vi "1_maximum_acceleration_main.vi"() -> ()   [LabVIEW 2019]
uses:
  Shared VIs/TypeDef_TDMS_States.ctl
  <vilib>/myRIO/Common/Instrument Driver Framework/myRIO v1.0/Encoder/typedefs/Encoder Signal Mode.ctl
  <vilib>/myRIO/Instrument Drivers/Onboard IO/AI/typedefs/AI Reference.ctl
  <vilib>/myRIO/Common/Instrument Driver Framework/Utilities/typedefs/myRIO Generic Hardware Reference.ctl
  <vilib>/myRIO/Common/Instrument Driver Framework/Utilities/typedefs/Hardware Version Enum.ctl
  <vilib>/myRIO/Common/Instrument Driver Framework/Utilities/typedefs/myRIO v1.0 Reference.ctl
  <vilib>/myRIO/Common/Instrument Driver Framework/Utilities/typedefs/Generic FPGA Reference.ctl
  <vilib>/myRIO/Common/Instrument Driver Framework/myRIO v1.0/AI/typedefs/AI Channels List.ctl
  <vilib>/myRIO/Common/Instrument Driver Framework/myRIO v1.0/AI/typedefs/AI Channels Enum.ctl
  <vilib>/myRIO/Common/Instrument Driver Framework/Utilities/typedefs/Analog Scaling Constants List.ctl
  <vilib>/myRIO/Common/Instrument Driver Framework/Utilities/typedefs/Analog Scaling Constants.ctl
  <vilib>/userDefined/High Color/nirio_resource_hc.ctl
  <vilib>/myRIO/Instrument Drivers/Onboard IO/AO/typedefs/AO Reference.ctl
  <vilib>/myRIO/Common/Instrument Driver Framework/myRIO v1.0/AO/typedefs/AO Channels List.ctl
  <vilib>/myRIO/Common/Instrument Driver Framework/myRIO v1.0/AO/typedefs/AO Channels Enum.ctl
  <vilib>/Platform/TimedLoop/XDataNode/timing_clust.ctl
  <vilib>/Platform/TimedLoop/XDataNode/nitl_modes.ctl
  <vilib>/Platform/TimedLoop/XDataNode/wakeup.ctl
  <vilib>/myRIO/Common/Instrument Driver Framework/myRIO v1.0/AI/vis/myRIO v1.1 Open AI.vi
  <vilib>/myRIO/Common/Instrument Driver Framework/myRIO v1.0/AO/vis/myRIO v1.1 Open AO.vi
  <vilib>/myRIO/Common/Instrument Driver Framework/Utilities/vis/Validate Channels.vi
  <vilib>/myRIO/Common/Instrument Driver Framework/myRIO v1.0/AI/vis/myRIO v1.0 Reserve AI.vi
  <vilib>/myRIO/Common/Instrument Driver Framework/myRIO v1.0/AO/vis/myRIO v1.0 Reserve AO.vi
  <vilib>/myRIO/Common/Instrument Driver Framework/myRIO v1.0/AI/vis/myRIO v1.0 Close AI.vi
  <vilib>/myRIO/Common/Instrument Driver Framework/myRIO v1.0/Encoder/vis/myRIO v1.0 Close Encoder.vi
  <vilib>/myRIO/Common/Instrument Driver Framework/myRIO v1.0/AO/vis/myRIO v1.0 Close AO.vi
  <vilib>/myRIO/Common/Instrument Driver Framework/myRIO v1.0/AI/vis/myRIO v1.0 Build MUX Configuration AI.vi
  <vilib>/myRIO/Common/Instrument Driver Framework/myRIO v1.0/Resource Manager/vis/myRIO v1.0 Reserve Channel List.vi
  <vilib>/myRIO/Common/Instrument Driver Framework/myRIO v1.0/AO/vis/myRIO v1.0 Build MUX Configuration AO.vi
  <vilib>/myRIO/Common/Instrument Driver Framework/myRIO v1.0/AI/vis/myRIO v1.0 Unreserve AI.vi
  <vilib>/myRIO/Common/Instrument Driver Framework/myRIO v1.0/Encoder/vis/myRIO v1.0 Unreserve Encoder.vi
  <vilib>/myRIO/Common/Instrument Driver Framework/myRIO v1.0/AO/vis/myRIO v1.0 Unreserve AO.vi
  <vilib>/myRIO/Common/Instrument Driver Framework/myRIO v1.0/Resource Manager/vis/myRIO v1.0 Reserve Channel.vi
  <vilib>/myRIO/Common/Instrument Driver Framework/myRIO v1.0/Resource Manager/vis/myRIO v1.0 Unreserve Channel.vi
  <vilib>/myRIO/Common/Instrument Driver Framework/myRIO v1.0/Resource Manager/vis/myRIO v1.0 Unreserve Channel List.vi
  <vilib>/myRIO/Common/Instrument Driver Framework/myRIO v1.0/Encoder/vis/myRIO v1.0 Build MUX Configuration Encoder.vi
  <vilib>/myRIO/Common/Instrument Driver Framework/myRIO v1.0/Resource Manager/vis/myRIO v1.0 Build Mutex Name.vi
  <vilib>/myRIO/Common/Instrument Driver Framework/myRIO v1.0/Resource Manager/vis/myRIO v1.0 Create Configuration List.vi
  <vilib>/Utility/VariantDataType/GetNumericInfo.vi
  <vilib>/Utility/error.llb/Error Cluster From Error Code.vi
  <vilib>/myRIO/Common/Instrument Driver Framework/myRIO v1.0/myRIO v1.1 Open.vi
  <vilib>/myRIO/Common/Instrument Driver Framework/myRIO v1.0/AO/vis/myRIO v1.0 Get Scaling Constants AO.vi
  <vilib>/myRIO/Common/Instrument Driver Framework/Utilities/vis/IO Manager.vi
  <vilib>/myRIO/Common/Instrument Driver Framework/Utilities/vis/Configuration Manager.vi
  <vilib>/myRIO/Common/Instrument Driver Framework/myRIO v1.0/myRIO v1.0 Close.vi
  <vilib>/myRIO/Common/Instrument Driver Framework/myRIO v1.0/AO/vis/myRIO v1.0 Write AO.vi
  <vilib>/myRIO/Common/Instrument Driver Framework/myRIO v1.0/AI/vis/myRIO v1.0 Get Scaling Constants AI.vi
  <vilib>/myRIO/Common/Instrument Driver Framework/myRIO v1.0/AI/vis/myRIO v1.0 Read AI.vi
  <vilib>/myRIO/Common/Instrument Driver Framework/myRIO v1.0/Encoder/vis/myRIO v1.0 Read Encoder.vi
  <vilib>/myRIO/Common/Instrument Driver Framework/myRIO v1.0/Encoder/vis/myRIO v1.0 Enable Encoder.vi
  <vilib>/myRIO/Common/Instrument Driver Framework/myRIO v1.0/Encoder/vis/myRIO v1.0 Shutdown Encoder.vi
  <vilib>/myRIO/Common/Instrument Driver Framework/myRIO v1.0/Resource Manager/vis/myRIO v1.0 Configure IO.vi
  <vilib>/myRIO/Instrument Drivers/Onboard IO/AO/vis/myRIO AO Open.xnode
  <vilib>/myRIO/Instrument Drivers/Onboard IO/AI/vis/myRIO AI Open.xnode
  <vilib>/Platform/TimedLoop/XDataNode/XDataNode.xnode
  <vilib>/myRIO/Instrument Drivers/Onboard IO/Encoder/Encoder.lvlib
  <vilib>/myRIO/Instrument Drivers/Onboard IO/AO/AO.lvlib
  <vilib>/Platform/TimedLoop/XDataNode/XDNodeRunTimeDep.lvlib
  <vilib>/myRIO/Instrument Drivers/Onboard IO/AI/AI.lvlib
panel:
  in  "TDMS Storage File Input":string
  out "TDMS States":T1
  in  "Save data?":bool
  in  "START":bool
  in  "Motor Input Voltage [V]":dbl
  out "Current (A)":dbl
  out "Loop Number (dt = 1 ms)":dbl
  in  "STOP":bool
  out "Elapsed Time (ms)":dbl
  out "Initial Time (ms)":dbl
  out "Encoder Position (deg)":dbl
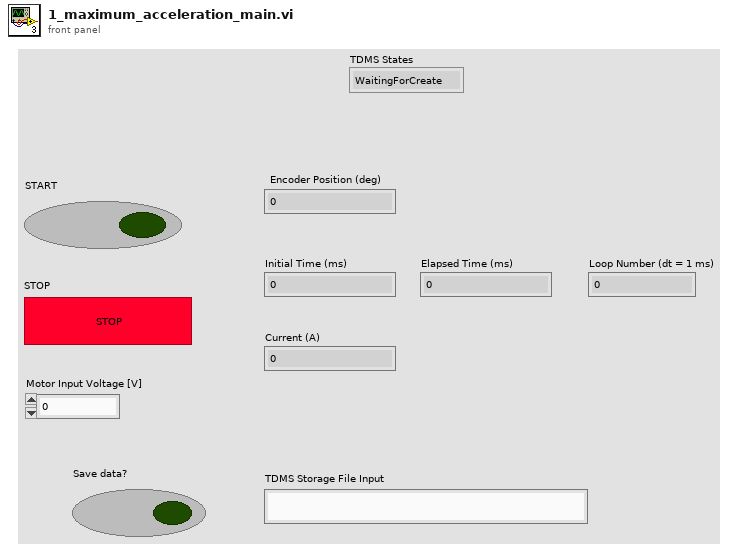
[diagram p1: front panel]
types:
  T1 = typedef "TypeDef_TDMS_States.ctl" = enum16{"WaitingForCreate", "Create", "Buffering", "Flushing", "Write", "Close"}
  T2 = typedef "nirio_resource_hc.ctl" = tag
  T3 = typedef "Hardware Version Enum.ctl" = enum16{"Unknown", "myRIO-1900", "myRIO-1950", "roboRIO", "NI ELVIS RIO CM", "ELVIS III"}
  T4 = enum16{"open", "open or create", "create or replace", "create", "open (read-only)"}
  T5 = typedef "XDNodeRunTimeDep.lvlib/timing_clust.ctl" = cluster{"Expected End [f-1]":u64, "Actual End [f-1]":u64, "Finished Late? [f-1]":bool, "Expected End [i-1]":u64, "Actual End [i-1]":u64, "Finished Late? [i-1]":bool, "Expected Start [i]":u64, "Actual Start [i]":u64, "Expected Start [f]":u64, "Actual Start [f]":u64, "Source Name":string, "Structure Name":string, "Period":i64, "Deadline":i64, "Offset":i64, "Start":i64, "Priority":i32, "Timeout":i32, "Mode":T6, "Wakeup Reason":T7, "Error":errorcluster, "Source Type":string, "Secondary Source Type":string, "Global End Time":u64, "Global Start Time":u64, "Frame Duration":u64, "Iteration Duration":u64, "Assigned CPU":i32, "I/O Scan Engine Mode":u32}
  T6 = typedef "XDNodeRunTimeDep.lvlib/nitl_modes.ctl" = enum32{"No Change", "Process missed periods, maintain original phase", "Discard missed periods, maintain original phase", "Process missed periods, ignore original phase", "Discard missed periods, ignore original phase"}
  T7 = typedef "XDNodeRunTimeDep.lvlib/wakeup.ctl" = enum32{"Normal", "Aborted", "Asynchronous wakeup", "Timing source error", "Timed loop error", "Timeout"}
  T8 = typedef "Encoder Signal Mode.ctl" = enum16{"Quadrature phase signal", "Step and direction signal"}
  T9 = typedef "AO.lvlib/AO Reference.ctl" = cluster{"myRIO Reference":T10, "AO Channel List":T13, "AO Scaling Constant List":T15}
  T10 = typedef "myRIO Generic Hardware Reference.ctl" = cluster{"myRIO Model":T3, "myRIO Hardware Reference":T11}
  T11 = typedef "myRIO v1.0 Reference.ctl" = cluster{"Generic FPGA Reference":T12, "Allow multiple opens":bool}
  T12 = typedef "Generic FPGA Reference.ctl" = refnum<k20>
  T13 = typedef "AO Channels List.ctl" = T14[]
  T14 = typedef "AO Channels Enum.ctl" = enum16{"Not Connected", "AudioOut/Left", "AudioOut/Right", "C/AO0", "C/AO1", "A/AO0", "A/AO1", "B/AO0", "B/AO1"}
  T15 = typedef "Analog Scaling Constants List.ctl" = T16[]
  T16 = typedef "Analog Scaling Constants.ctl" = cluster{"LSB Weight (Volts)":dbl, "Offset (Volts)":dbl, "Signed?":bool}
  T17 = typedef "AI.lvlib/AI Reference.ctl" = cluster{"myRIO Reference":T10, "AI Channels List":T18, "AI Scaling Constants List":T15}
  T18 = typedef "AI Channels List.ctl" = T19[]
  T19 = typedef "AI Channels Enum.ctl" = enum16{"Not Connected", "AudioIn/Left", "AudioIn/Right", "C/AI0", "C/AI1", "A/AI0", "A/AI1", "A/AI2", "A/AI3", "A/AI4", "A/AI5", "A/AI6", "A/AI7", "B/AI0", "B/AI1", "B/AI2", "B/AI3", "B/AI4", "B/AI5", "B/AI6", "B/AI7", "AI/AI0", "AI/AI1", "AI/AI2", "AI/AI3", "A/AI0 (DIFF)", "A/AI1 (DIFF)", "A/AI2 (DIFF)", "A/AI3 (DIFF)", "B/AI0 (DIFF)", "B/AI1 (DIFF)", "B/AI2 (DIFF)", "B/AI3 (DIFF)"}
  T20 = typedef "Encoder.lvlib/Encoder Reference.ctl" = cluster{"myRIO Reference":T10, "Encoder Channels Enum":T21}
  T21 = typedef "Encoder Channels Enum.ctl" = enum16{"Not Connected", "C/ENC0", "C/ENC1", "A/ENC", "A/ENC0", "A/ENC1", "A/ENC2", "A/ENC3", "A/ENC4", "A/ENC5", "A/ENC6", "A/ENC7", "A/ENC8", "A/ENC9", "B/ENC", "B/ENC0", "B/ENC1", "B/ENC2", "B/ENC3", "B/ENC4", "B/ENC5", "B/ENC6", "B/ENC7", "B/ENC8", "B/ENC9", "DIO/ENC0", "DIO/ENC1", "DIO/ENC2", "DIO/ENC3", "DIO/ENC4"}
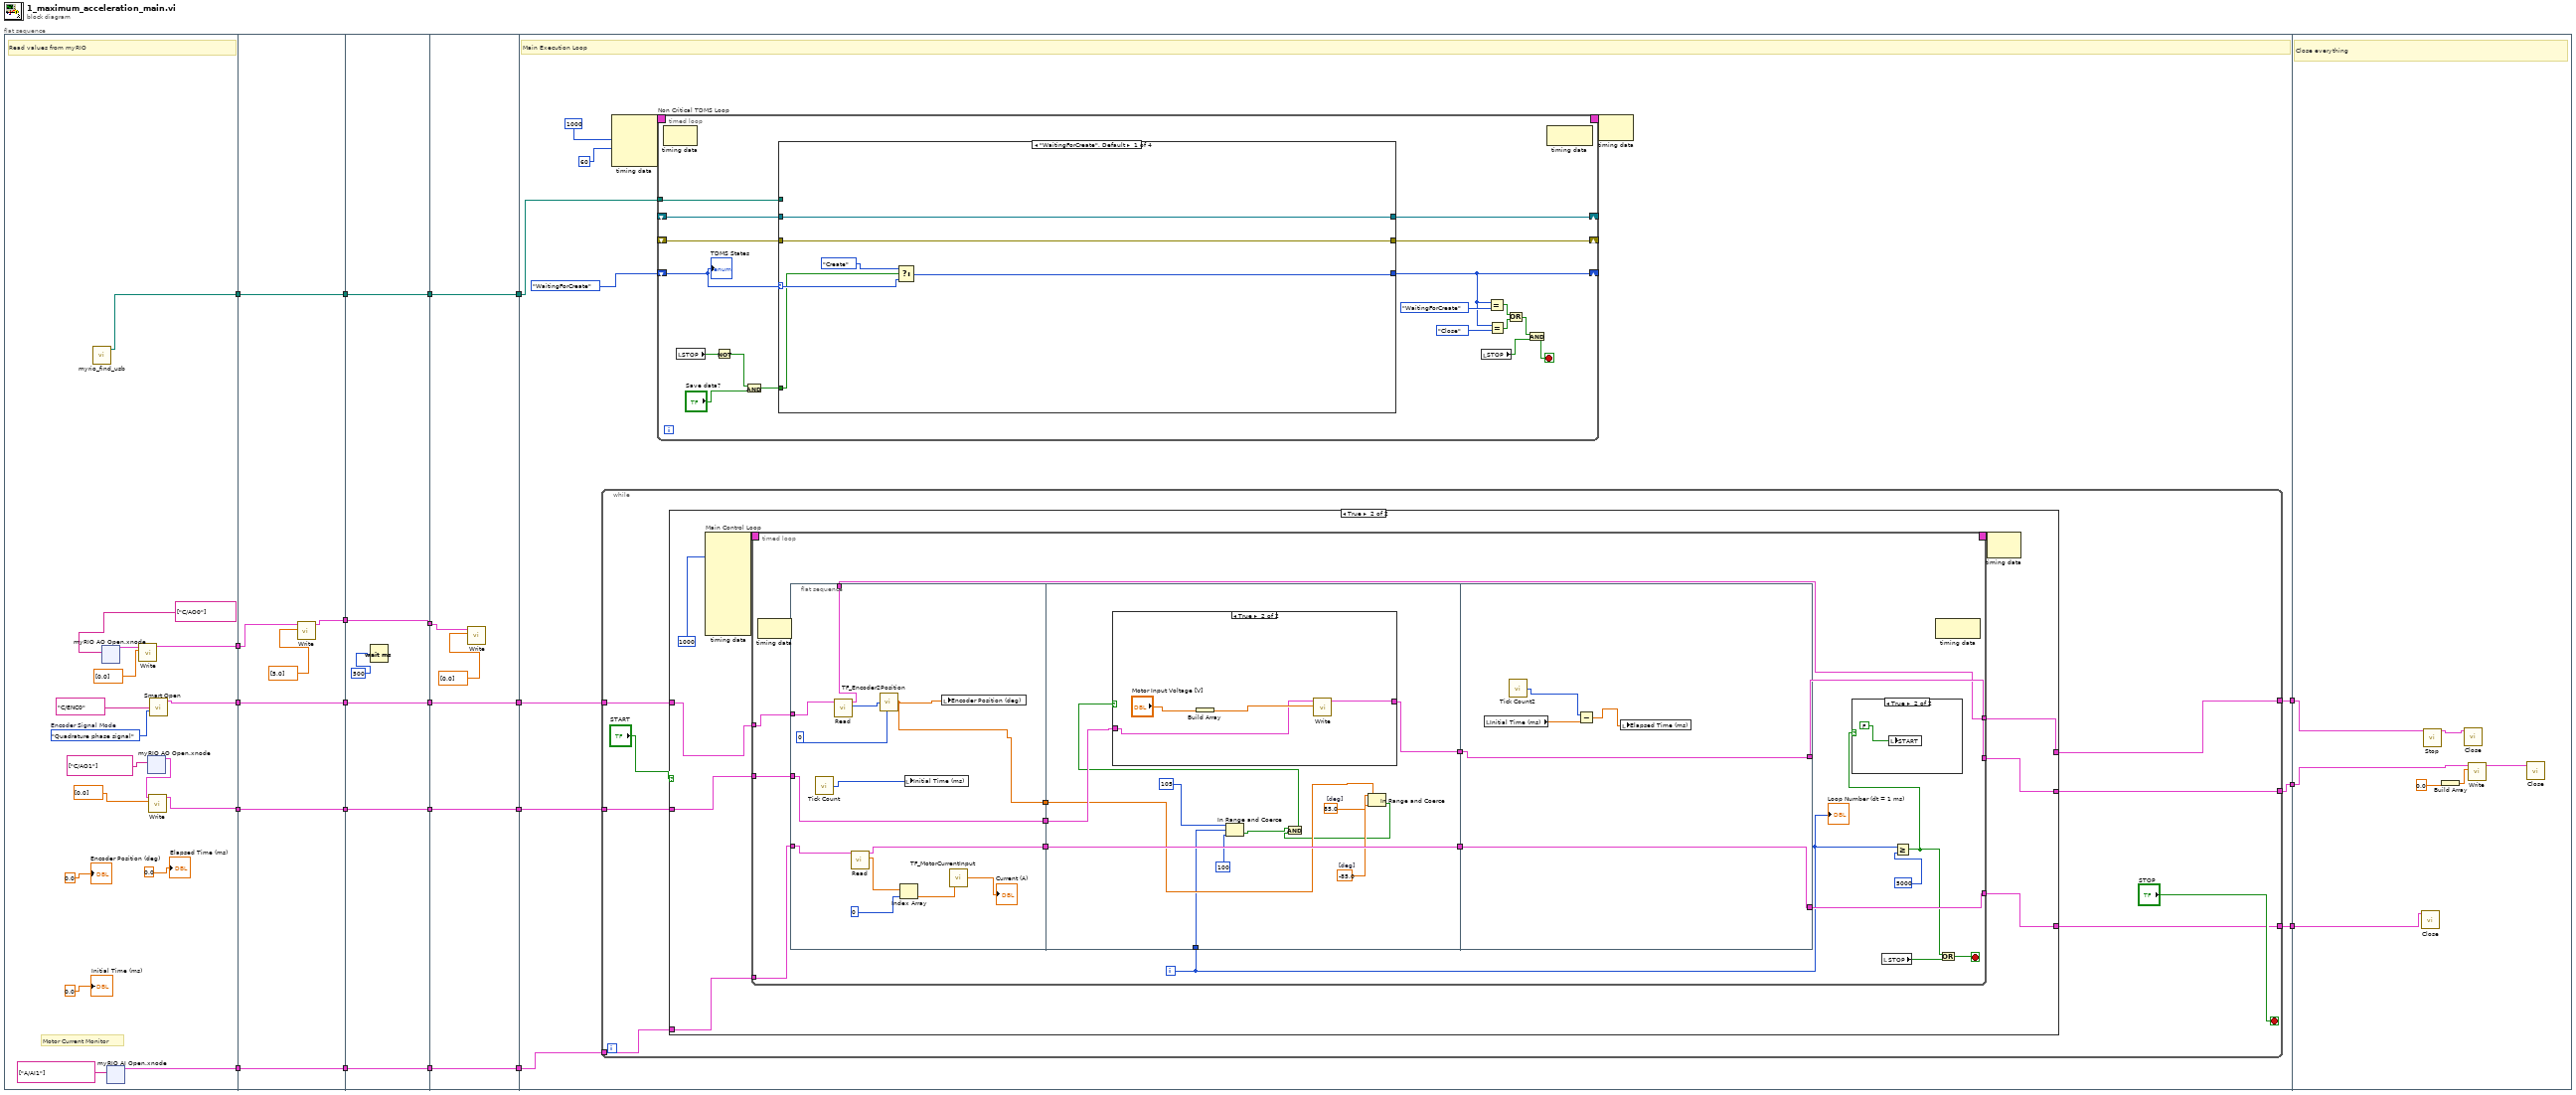
[diagram p0: block diagram]
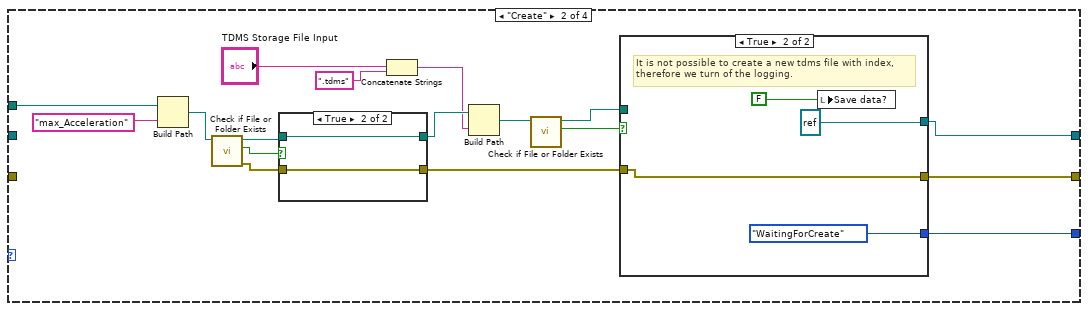
[diagram p2: hidden frame]
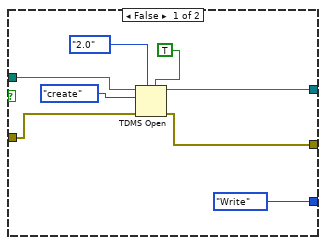
[diagram p3: hidden frame]
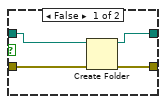
[diagram p4: hidden frame]
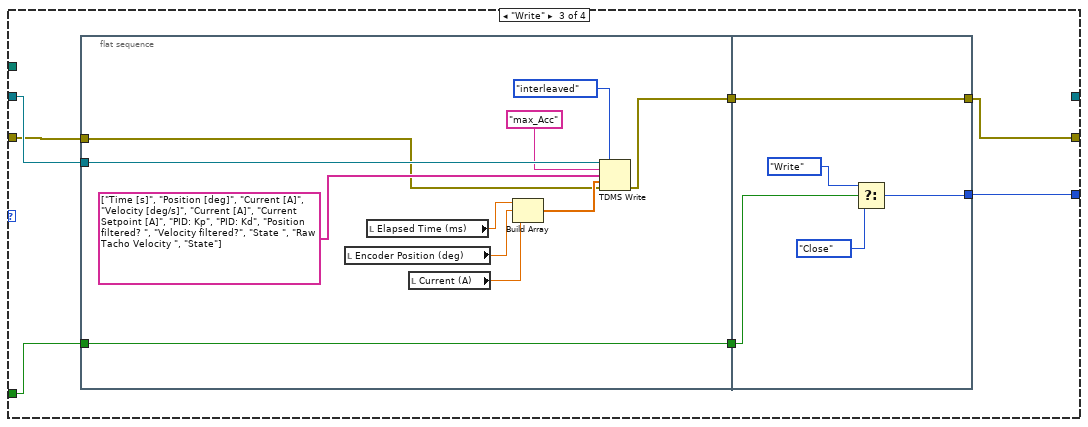
[diagram p5: hidden frame]
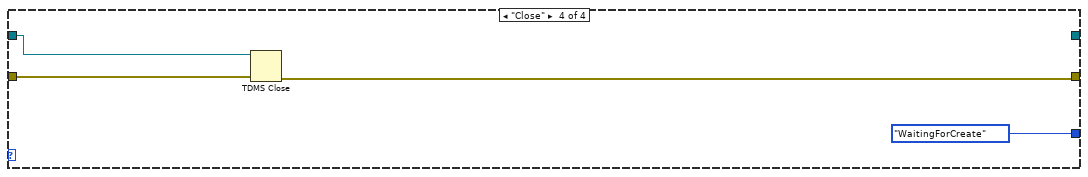
[diagram p6: hidden frame]
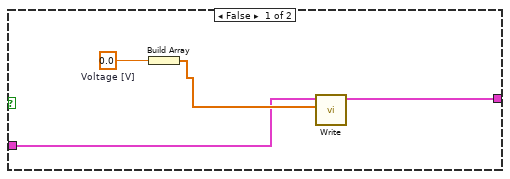
[diagram p9: hidden frame]
diagram:
  n1 = flat-sequence {
    tunnel: [w31] -> w15
    tunnel: [w30] -> w13
    tunnel: [w26] -> w11
    tunnel: [w24] -> w6
    tunnel: [w23] -> w1
    tunnel: w15 -> [w100]
    tunnel: [w100] -> w14
    tunnel: w13 -> [w99]
    tunnel: [w99] -> w12
    tunnel: w11 -> [w97]
    tunnel: [w96] -> w10
    tunnel: [w95] -> w7
    tunnel: w6 -> [w95]
    tunnel: [w94] -> w2
    tunnel: w1 -> [w94]
    tunnel: w14 -> [w106]
    tunnel: [w106] -> w20
    tunnel: w12 -> [w105]
    tunnel: [w105] -> w18
    tunnel: [w103] -> w16
    tunnel: w10 -> [w103]
    tunnel: [w102] -> w8
    tunnel: w7 -> [w102]
    tunnel: [w101] -> w3
    tunnel: w2 -> [w101]
    tunnel: w20 -> [w112]
    tunnel: [w112] -> w19
    tunnel: w18 -> [w111]
    tunnel: [w111] -> w17
    tunnel: w16 -> [w110]
    tunnel: [w108] -> w9
    tunnel: w8 -> [w108]
    tunnel: [w107] -> w4
    tunnel: w3 -> [w107]
    tunnel: w19 -> [w123]
    tunnel: w17 -> [w124]
    tunnel: [w121] -> w22
    tunnel: [w122] -> w21
    tunnel: w9 -> [w120]
    tunnel: [w119] -> w5
    tunnel: w4 -> [w113]
    tunnel: w22 -> [w301]
    tunnel: w21 -> [w300]
    tunnel: w5 -> [w299]
    frame #0 {
      w38 = Encoder_Signal_Mode."Quadrature phase signal"  # Encoder Signal Mode
      # "Motor Current Monitor"
      # "Read values from myRIO"
      n2 = call "myrio_find_usb.vi"() -> ("Largest USB Partition Path"=w23:path)  [unwired: 9 in, 2 out]
      n3 = xnode "myRIO AO Open.xnode"("Channel Names"=tag[] ["C/AO0"]) -> ("AO Ref Out"=w29:T9)  [unwired: 2 in, 1 out]
      n4 = xnode "myRIO AI Open.xnode"("Channel Names"=tag[] ["A/AI1"]) -> ("AI Ref Out"=w24:T17)  [unwired: 2 in, 1 out]
      n5 = call <vilib>:"Write.vi"("Values"=dbl[] [0.0], "AO Ref In"=w29) -> ("AO Ref Out"=w26:T9)  [unwired: 7 in, 1 out]
      n6 = xnode "myRIO AO Open.xnode"("Channel Names"=tag[] ["C/AO1"]) -> ("AO Ref Out"=w36:T9)  [unwired: 2 in, 1 out]
      n7 = call <vilib>:"Write.vi"("Values"=dbl[] [0.0], "AO Ref In"=w36) -> ("AO Ref Out"=w30:T9)  [unwired: 7 in, 1 out]
      n8 = call <vilib>:"Smart Open.vi"("Encoder Signal Mode"=w38, "Channel Name"=tag "C/ENC0") -> ("Encoder Ref Out"=w31:T20)  [unwired: 8 in, 1 out]
      "Encoder Position (deg)" <- 0.0
      "Initial Time (ms)" <- 0.0
      "Elapsed Time (ms)" <- 0.0
    }
    frame #1 {
      n9 = call <vilib>:"Write.vi"("Values"=dbl[] [5.0], "AO Ref In"=w97) -> ("AO Ref Out"=w96:T9)  [unwired: 7 in, 1 out]
    }
    frame #2 {
      n10 = Wait (ms)(milliseconds to wait=500) -> ()  [unwired: 1 out]
    }
    frame #3 {
      n11 = call <vilib>:"Write.vi"("Values"=dbl[] [0.0], "AO Ref In"=w110) -> ()  [unwired: 7 in, 2 out]
    }
    frame #4 {
      # "Main Execution Loop"
      n12 = while {
        tunnel: w124 -> [w225]
        tunnel: w123 -> [w224]
        tunnel: [w221] -> w122
        tunnel: [w222] -> w121
        tunnel: w120 -> [w220]
        tunnel: [w219] -> w119
        stop <- "STOP" stop-if-true
        n13 = case shown="True" "START" {
          tunnel: w225 -> [w227 w234]
          tunnel: w224 -> [w228 w233]
          tunnel: [w227 w232] -> w222
          tunnel: [w228 w231] -> w221
          tunnel: w220 -> [w226 w230]
          tunnel: [w226 w229] -> w219
          frame False {
          }
          frame True {
            n14 = node-c288(1000) -> (w237:T5)  [unwired: 9 in]
            n15 = timed-loop "Main Control Loop" {
              timing: w237 -> [_]
              timing-out: [_] -> w236
              tunnel: w233 -> [w253]
              tunnel: w234 -> [w252]
              tunnel: [w249] -> w232
              tunnel: [w248] -> w231
              tunnel: w230 -> [w247]
              tunnel: [w244] -> w229
              i -> [w242]
              stop <- w240 stop-if-true
              n16 = node-c288() -> ()  [unwired: 1 in, 1 out]
              n17 = flat-sequence {
                tunnel: w253 -> [w265]
                tunnel: w252 -> [w264]
                tunnel: [w264] -> w251
                tunnel: [w263] -> w248
                tunnel: w247 -> [w261]
                tunnel: [w256] -> w245
                tunnel: [w255] -> w243
                tunnel: w242 -> [w269]
                tunnel: w251 -> [w279]
                tunnel: [w278] -> w250
                tunnel: [w277] -> w246
                tunnel: w245 -> [w277]
                tunnel: w243 -> [w274]
                tunnel: w250 -> [w290]
                tunnel: [w290] -> w249
                tunnel: [w288] -> w244
                tunnel: w246 -> [w288]
                frame #0 {
                  n18 = call "Tick Count"() -> ("Tick Count(mSec)"=w262:u32)
                  n19 = call <vilib>:"Read.vi"("Encoder Ref In"=w265) -> ("Counter Value"=w267:i32, "Encoder Ref Out"=w263:T20)  [unwired: 6 in, 3 out]
                  n20 = call <vilib>:"Read.vi"("AI Ref In"=w261) -> ("Values"=w260:dbl[], "AI Ref Out"=w256:T17)  [unwired: 8 in, 1 out]
                  n21 = call "TF_Encoder2Position.vi"("Counter Value"=w267, "Offset"=0) -> ("Position [deg]"=w255:dbl)  [unwired: 3 in]
                  n22 = Index Array(array=w260, index=0) -> (element=w258:dbl)
                  n23 = local write "Initial Time (ms)"(w262) -> ()
                  n24 = local write "Encoder Position (deg)"(w255) -> ()
                  n25 = call "TF_MotorCurrentInput.vi"("Motor Current Monitor Value [V]"=w258) -> ("Current [A]"=→"Current (A)":dbl)
                }
                frame #1 {
                  w275 = 85.0  # [deg]
                  w276 = -85.0  # [deg]
                  n26 = In Range and Coerce(upper limit=105, x=w269, lower limit=100) -> (In Range?=w268:bool)  [unwired: 1 out]
                  n27 = In Range and Coerce(upper limit=w275, x=w274, lower limit=w276) -> (In Range?=w272:bool)  [unwired: 1 out]
                  n28 = And(x=w268, y=w272) -> (x .and. y?=w273:bool)
                  n29 = case shown="True" w273 {
                    tunnel: w279 -> [w281 w286]
                    tunnel: [w280 w285] -> w278
                    frame False {
                      w282 = 0.0  # Voltage [V]
                      n30 = Build Array(w282) -> (w283:dbl[])
                      n31 = call <vilib>:"Write.vi"("Values"=w283, "AO Ref In"=w281) -> ("AO Ref Out"=w280:T9)  [unwired: 7 in, 1 out]
                    }
                    frame True {
                      n32 = Build Array("Motor Input Voltage [V]") -> (w287:dbl[])
                      n33 = call <vilib>:"Write.vi"("Values"=w287, "AO Ref In"=w286) -> ("AO Ref Out"=w285:T9)  [unwired: 7 in, 1 out]
                    }
                  }
                }
                frame #2 {
                  n34 = local read "Initial Time (ms)"() -> (w292:dbl)
                  n35 = call "Tick Count2"() -> ("Tick Count(mSec)"=w289:u32)
                  n36 = Subtract(x=w289, y=w292) -> (x-y=w291:dbl)
                  n37 = local write "Elapsed Time (ms)"(w291) -> ()
                }
              }
              n38 = local read "STOP"() -> (w239:bool)
              n39 = Greater Or Equal?(x=w242, y=5000) -> (x >= y?=w238:bool)
              n40 = case shown="True" w238 {
                frame False {
                }
                frame True {
                  n41 = local write "START"(FALSE) -> ()
                }
              }
              n42 = node-c288() -> ()  [unwired: 1 in, 1 out]
              n43 = Or(x=w238, y=w239) -> (x .or. y?=w240:bool)
              "Loop Number (dt = 1 ms)" <- w242
            }
            n44 = node-c288(w236) -> ()  [unwired: 1 out]
          }
        }
      }
      n45 = node-c288(1000, 60) -> (w118:T5)  [unwired: 2 in]
      n46 = timed-loop "Non Critical TDMS Loop" {
        timing: w118 -> [_]
        timing-out: [_] -> w117
        shift-right: [w130] -> _
        shift-left: TypeDef_TDMS_States."WaitingForCreate" ("TDMS States") -> [w137]
        tunnel: w113 -> [w142]
        shift-right: [w141] -> _
        shift-left: _ -> [w139]
        shift-right: [w140] -> _
        shift-left: _ -> [w138]
        stop <- w126 stop-if-true
        n47 = node-c288() -> ()  [unwired: 1 in, 1 out]
        n48 = local read "STOP"() -> (w136:bool)
        n49 = Not(x=w136) -> (.not. x?=w134:bool)
        n50 = And(x=w134, y="Save data?") -> (x .and. y?=w135:bool)
        n51 = case shown="\"WaitingForCreate\", Default" w137 {
          selector: w137 -> [w147 _ _ _]
          tunnel: [w146 w149 w188 TypeDef_TDMS_States."WaitingForCreate" ("TDMS States")] -> w130
          tunnel: w142 -> [_ w165 _ _]
          tunnel: [w144 w152 w184 w208] -> w141
          tunnel: [w143 w150 _ _] -> w140
          tunnel: w138 -> [w143 _ w190 w210]
          tunnel: w139 -> [w144 _ w189 w209]
          tunnel: w135 -> [w145 _ w186 _]
          frame "WaitingForCreate", Default {
            n52 = Select(t=TypeDef_TDMS_States."Create" ("TDMS States"), s=w145, f=w147) -> (s? t:f=w146:T1)
          }
          frame "Create" {
            n53 = Build Path(base path=w165, name or relative path="max_Acceleration") -> (appended path=w161:path)
            n54 = call <vilib>:"Check if File or Folder Exists.vi"("path"=w161) -> ("error out"=w158:errorcluster, "file or folder exists?"=w160:bool, "dup path"=w159:path)  [unwired: 8 in]
            n55 = case shown="True" w160 {
              tunnel: w159 -> [w181 w182]
              tunnel: [w180 w183] -> w153
              tunnel: w158 -> [w179 w183]
              tunnel: [w178 w182] -> w157
              frame False {
                n56 = Create Folder(path (use dialog)=w181, error in=w179) -> (created path=w178:path, error out=w180:errorcluster)  [unwired: 1 in, 1 out]
              }
              frame True {
              }
            }
            n57 = Concatenate Strings("TDMS Storage File Input", ".tdms") -> (w156:string)
            n58 = Build Path(base path=w157, name or relative path=w156) -> (appended path=w155:path)
            n59 = call <vilib>:"Check if File or Folder Exists.vi"("path"=w155) -> ("file or folder exists?"=w154:bool, "dup path"=w151:path)  [unwired: 8 in, 1 out]
            n60 = case shown="True" w154 {
              tunnel: w153 -> [w173 w177]
              tunnel: [w172 w177] -> w152
              tunnel: w151 -> [w170 _]
              tunnel: [w169 refnum<k34> refnum ("tdms file out")] -> w150
              tunnel: [TypeDef_TDMS_States."Write" ("TDMS States") TypeDef_TDMS_States."WaitingForCreate" ("TDMS States")] -> w149
              frame False {
                n61 = TDMS Open(5:TRUE, 7:enum16{"1.0", "2.0"}."2.0" ("file format version (2.0)"), 8:w173, 10:T4."create" ("operation (0:open)"), 11:w170) -> (0:w172:errorcluster, 3:w169:refnum<k34>)  [unwired: 2 in]
              }
              frame True {
                # "It is not possible to create a new tdms file with index,\ntherefore we turn of the logging."
                n62 = local write "Save data?"(FALSE ("Save data?")) -> ()
              }
            }
          }
          frame "Write" {
            n63 = flat-sequence {
              tunnel: w190 -> [w198]
              tunnel: w189 -> [w194]
              tunnel: [w193] -> w187
              tunnel: w186 -> [w193]
              tunnel: [w192] -> w185
              tunnel: [w204] -> w188
              tunnel: w187 -> [w203]
              tunnel: w185 -> [w202]
              tunnel: [w202] -> w184
              frame #0 {
                n64 = local read "Encoder Position (deg)"() -> (w200:dbl)
                n65 = local read "Elapsed Time (ms)"() -> (w201:dbl)
                n66 = local read "Current (A)"() -> (w199:dbl)
                n67 = Build Array(w201, w200, w199) -> (w195:dbl[])
                n68 = TDMS Write(0:w198, 1:enum16{"decimated", "interleaved"}."interleaved" ("data layout (0:decimated)"), 5:"max_Acc" ("group name in (Untitled)"), 7:string[] ["Time [s]", "Position [deg]", "Current [A]", "Velocity [deg/s]", "Current [A]", "Current Setpoint [A]", "PID: Kp", "PID: Kd", "Position filtered? ", "Velocity filtered?", "State ", "Raw Tacho Velocity ", "State"], 9:w195, 11:w194) -> (15:w192:errorcluster)  [unwired: 3 out]
              }
              frame #1 {
                n69 = Select(t=TypeDef_TDMS_States."Write" ("TDMS States"), s=w203, f=TypeDef_TDMS_States."Close" ("TDMS States")) -> (s? t:f=w204:T1)
              }
            }
          }
          frame "Close" {
            n70 = TDMS Close(8:w209, 11:w210) -> (0:w208:errorcluster)  [unwired: 1 out]
          }
        }
        n71 = local read "STOP"() -> (w125:bool)
        n72 = Equal?(x=w130, y=TypeDef_TDMS_States."WaitingForCreate" ("TDMS States")) -> (x = y?=w129:bool)
        n73 = Equal?(x=w130, y=TypeDef_TDMS_States."Close" ("TDMS States")) -> (x = y?=w128:bool)
        n74 = Or(x=w129, y=w128) -> (x .or. y?=w127:bool)
        n75 = And(x=w127, y=w125) -> (x .and. y?=w126:bool)
        n76 = node-c288() -> ()  [unwired: 1 in, 1 out]
        "TDMS States" <- w137
      }
      n77 = node-c288(w117) -> ()  [unwired: 1 out]
    }
    frame #5 {
      # "Close everything"
      n78 = call <vilib>:"Close.vi"("AI Ref In"=w299) -> ()  [unwired: 10 in, 1 out]
      n79 = call <vilib>:"Stop.vi"("Encoder Ref In"=w300) -> ("Encoder Ref Out"=w305:T20)  [unwired: 9 in, 1 out]
      n80 = Build Array(0.0) -> (w302:dbl[])
      n81 = call <vilib>:"Close.vi"("Encoder Ref In"=w305) -> ()  [unwired: 10 in, 1 out]
      n82 = call <vilib>:"Write.vi"("Values"=w302, "AO Ref In"=w301) -> ("AO Ref Out"=w304:T9)  [unwired: 7 in, 1 out]
      n83 = call <vilib>:"Close.vi"("AO Ref In"=w304) -> ()  [unwired: 10 in, 1 out]
    }
  }
